vi "Util - Get Drive Letters.vi"(8 "Error In":errorcluster) -> (0 "Error Out":errorcluster, 3 "Drive Letters":string[](array[string]))   [LabVIEW 2020]
doc: "Author: Erich Schlieper\n\nUses the command line to get a string of all the drives that are connected to the computer this VI is run on. The string of drive letters is then transformed into an array of drive letters output in the <B>Drive Letters</B> output."
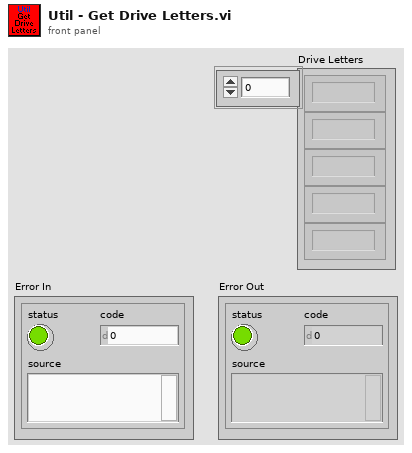
[diagram p1: front panel]
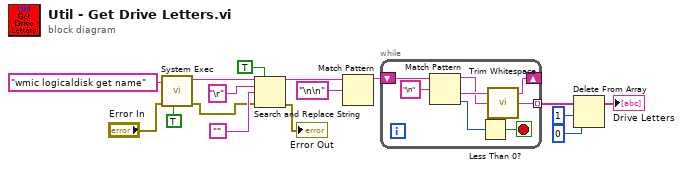
[diagram p0: block diagram]
diagram:
  n1 = call <vilib>:"System Exec.vi"("run minimized? (F)"=TRUE, "error in (no error)"="Error In", "command line"="wmic logicaldisk get name") -> ("error out"=w2:errorcluster, "standard output"=w14:string)  [unwired: 5 in, 2 out]
  n2 = Search and Replace String(replace all?=TRUE ("replace all? (F)"), input string=w14, search string="\r" ("substring (\"\")"), replace string="", error in=w2) -> (result string=w6:string, error out=→"Error Out":errorcluster)  [unwired: 3 in, 2 out]
  n3 = Match Pattern(string=w6, regular expression="\n\n") -> (before substring=w4:string)  [unwired: 1 in, 3 out]
  n4 = while {
    shift-right: [w21] -> _
    shift-left: w4 -> [w23]
    tunnel: [w17] -> w10 mode=indexing
    stop <- w18 stop-if-true
    n5 = Match Pattern(string=w23, regular expression="\n") -> (before substring=w20:string, after substring=w21:string, offset past match=w19:i32)  [unwired: 1 in, 1 out]
    n6 = Less Than 0?(x=w19) -> (x < 0?=w18:bool)
    n7 = call <vilib>:"Trim Whitespace.vi"("string"=w20) -> ("trimmed string"=w17:string)  [unwired: 1 in]
  }
  n8 = Delete From Array(array=w10, length=1, index=0) -> (array with subset deleted=→"Drive Letters":string[])  [unwired: 1 out]
